vi "lookup_table_and_invert.vi"() -> ()   [LabVIEW 2020]
doc: "VI che calcola l'istogramma dell'immagine"
uses:
  <vilib>/vision/NI_Vision_Development_Module.lvlib
panel:
  in  "Tab Control":enum32{"Immagini", "Istogrammi"}(tab)
  out "Gray level image":T1(plugin-control)
  out "Lookup":T1(plugin-control)
  in  "Operator":T2(ring)
  out "Invert":T1(plugin-control)
  in  "stop":bool
  in  "X Value":sgl format="%.2f"
  in  "Path Image Load":path
  in  "error in (no error)":errorcluster
  out "error out":errorcluster
  out "Istogramma":T3(graph)
  out "Istogramma Lookup":T3(graph)
  out "Istogramma Invert":T3(graph)
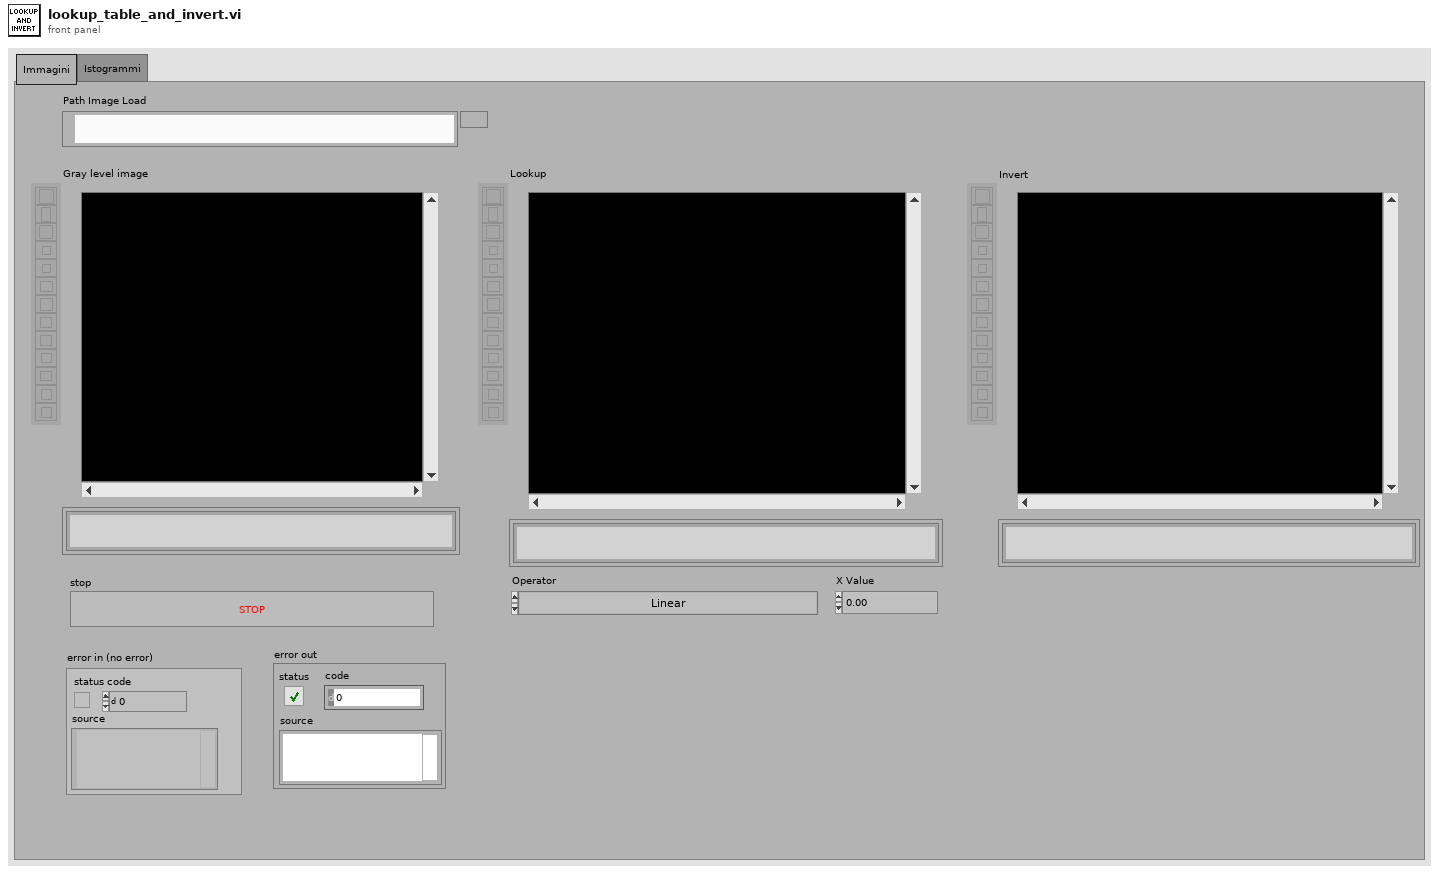
[diagram p1: front panel]
types:
  T1 = typedef "IMAQ Image.ctl" = refnum<image>
  T2 = enum32{"Linear", "Log", "Exp", "Square", "Square root", "Power X", "Power 1/X"}
  T3 = cluster{"Starting Value":sgl, "Incremental Value":sgl, "Histogram":u32[]}
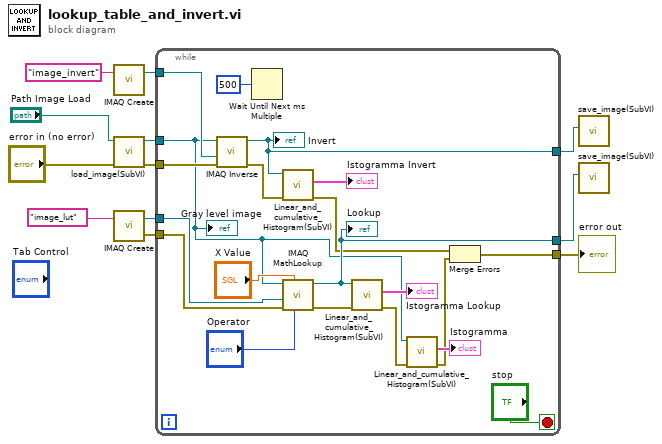
[diagram p0: block diagram]
diagram:
  n1 = call "IMAQ Create"("Image Name"="image_invert") -> ("New Image"=w11:T1)  [unwired: 4 in, 1 out]
  n2 = call "load_image(SubVI).vi"("error in (no error)"="error in (no error)", "Image Path"="Path Image Load") -> ("error out"=w3:errorcluster, "Image GRAY"=w4:T1)  [unwired: 8 in]
  n3 = call "IMAQ Create"("Image Name"="image_lut") -> ("New Image"=w9:T1, "error out"=w8:errorcluster)  [unwired: 4 in]
  n4 = while {
    tunnel: w11 -> [w29]
    tunnel: w4 -> [w20]
    tunnel: w3 -> [w27]
    tunnel: w9 -> [w26]
    tunnel: w8 -> [w25]
    tunnel: [w24] -> w7
    tunnel: [w23] -> w2
    tunnel: [w16] -> w1
    stop <- "stop" stop-if-true
    n5 = call "IMAQ Inverse"("error in (no error)"=w27, "Image Dst"=w29, "Image Src"=w20) -> ("error out"=w15:errorcluster, "Image Dst Out"=w16:T1)  [unwired: 7 in]
    "Invert" <- w16
    n6 = Wait Until Next ms Multiple(millisecond multiple=u32 500) -> ()  [unwired: 1 out]
    n7 = call "Linear_and_cumulative_Histogram(SubVI).vi"("error in (no error)"=w15, "Image GRAY"=w16) -> ("error out"=w14:errorcluster, "Linear Histogram"=→"Istogramma Invert":T3)  [unwired: 7 in, 1 out]
    n8 = call "IMAQ MathLookup"("Operator"="Operator", "X Value"="X Value", "error in (no error)"=w25, "Image Dst"=w26, "Image Src"=w20) -> ("error out"=w21:errorcluster, "Image Dst Out"=w23:T1)  [unwired: 5 in]
    "Lookup" <- w23
    n9 = call "Linear_and_cumulative_Histogram(SubVI).vi"("error in (no error)"=w21, "Image GRAY"=w23) -> ("error out"=w18:errorcluster, "Linear Histogram"=→"Istogramma Lookup":T3)  [unwired: 7 in, 1 out]
    n10 = call "Linear_and_cumulative_Histogram(SubVI).vi"("error in (no error)"=w18, "Image GRAY"=w20) -> ("error out"=w17:errorcluster, "Linear Histogram"=→"Istogramma":T3)  [unwired: 7 in, 1 out]
    n11 = Merge Errors(w14, w17) -> (w24:errorcluster)
    "Gray level image" <- w20
  }
  "error out" <- w7
  n12 = call "save_image(SubVI).vi"("Image"=w1) -> ()  [unwired: 9 in, 2 out]
  n13 = call "save_image(SubVI).vi"("Image"=w2) -> ()  [unwired: 9 in, 2 out]
